vi "initial-Pos.vi"(8 "error in (no error)":errorcluster) -> (0 "error out":errorcluster)   [LabVIEW 2014]
doc: "André Romero - 2023\nandretec@ifsc.usp.br\nIFSC - USP"
uses:
  Global Motors.vi
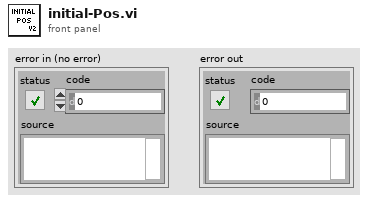
[diagram p1: front panel]
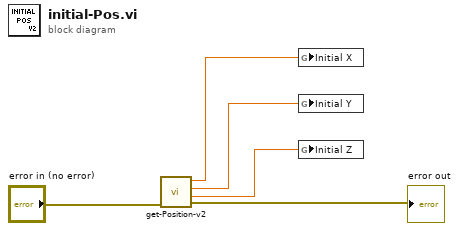
[diagram p0: block diagram]
diagram:
  n1 = call "get-Position-v2.vi"("error in (no error)"="error in (no error)") -> ("error out"=→"error out":errorcluster, "Position Z"=w2:sgl, "Position Y"=w3:dbl, "Position X"=w1:dbl)  [unwired: 7 in]
  n2 = global write "Global Motors.vi" "Initial X"(w1) -> ()
  n3 = global write "Global Motors.vi" "Initial Y"(w3) -> ()
  n4 = global write "Global Motors.vi" "Initial Z"(w2) -> ()
